vi "Dut Post Initiate.vi"(8 "error in (no error)":errorcluster, 11 "MTK7615 in":refnum<class "MTK7615.lvclass">) -> (0 "error out":errorcluster, 3 "MTK7615 out":refnum<class "MTK7615.lvclass">)   [LabVIEW 2015, in "MTK7615.lvlib" / "MTK7615.lvclass"]
uses:
  MTK7615.lvclass
  Technologies/WLAN/Dut/Objects/BASE_class/niDTS WLAN Dut.lvclass
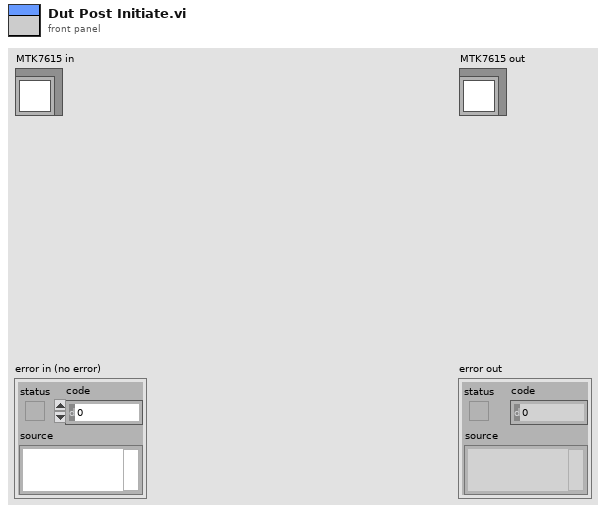
[diagram p1: front panel]
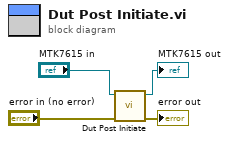
[diagram p0: block diagram]
diagram:
  n1 = call-parent "Dut Post Initiate.vi"("error in (no error)"="error in (no error)", "niDTS Dut in"="MTK7615 in") -> ("error out"=→"error out":errorcluster, "niDTS Dut out"=→"MTK7615 out":refnum<class "MTK7615.lvclass">)  [unwired: 8 in]
